vi "NotifyLvFPGACompileFinish.vi"() -> ()   [LabVIEW 2013]
uses:
  <vilib>/Utility/sysdir.llb/System Directory Type.ctl
  <vilib>/Utility/miscctls.llb/LVPointTypeDef.ctl
  <vilib>/ptbypt/NI_PtbyPt.lvlib
panel:
  out "title":string="NotifyLvFPGACompileFinish"
  in  "Prohibit time":T1
  out "smtp error msg":string
  in  "Interval_sec":i32=60
  in  "SendTo":T2
  in  "SMTP Setting":T3={"smtp server"="", "From"="", "port number"=25, "chk smtp auth"=FALSE, "userID"="", "password"="", "chk ssl"=FALSE}
  in  "Tab":enum32{"Log"}(tab)
  out "Log":string
  out "コンパイル中":bool
  out "Compile FPGA-Target":string
  out "MailBody":string
  in  "Btn SendMail":bool
  out "Compile Folder":path
  out "flag Compiling":bool
  out "監視中":bool
  out "flag Monitoring":bool
  in  "FPGA Compile path":path=path "C:/NIFPGA/compilation"
  in  "Btn Settings":bool
  in  "Btn Stop":bool
  in  "Btn Start":bool
  # "FPGAコンパイル終了時に\n指定したメールアドレスに\n結果メールを送信します。"
  # "FPGA モジュールがインストールされているPCで実行してください。"
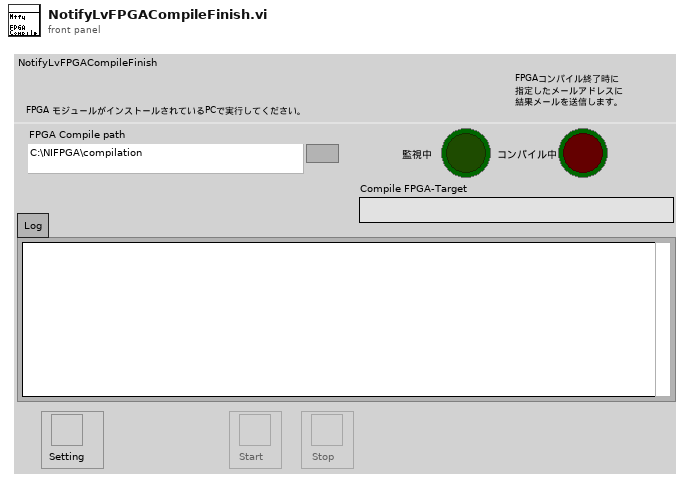
[diagram p1: front panel]
types:
  T1 = cluster{"chk enable":bool, "start hour":u8, "end hour":u8}
  T2 = cluster{"To 1":cluster{"chk":bool, "To":string}, "To 2":cluster{"chk":bool, "To":string}, "To 3":cluster{"chk":bool, "To":string}}
  T3 = cluster{"smtp server":string, "From":string, "port number":i32, "chk smtp auth":bool, "userID":string, "password":string, "chk ssl":bool}
  T4 = typedef "System Directory Type.ctl" = i32
  T5 = enum8{"Enabled", "Disabled", "Disabled and Grayed Out"}
  T6 = cluster{"SMTP Setting out":cluster{"smtp server":string, "From":string, "port number":i32, "chk smtp auth":bool, "userID":string, "password":string, "chk ssl":bool}, "SendTo out":cluster{"To 1":cluster{"chk":bool, "To":string}, "To 2":cluster{"chk":bool, "To":string}, "To 3":cluster{"chk":bool, "To":string}}, "Prohibit time out":cluster{"chk enable":bool, "start hour":u8, "end hour":u8}}
  T7 = typedef "LVPointTypeDef.ctl" = cluster{"Horizontal":i16, "Vertical":i16}
  T8 = cluster{bool, "include Ctrl key?":bool, string}[]
  T9 = cluster{"配列[0]":i16, "配列[1]":i16, "配列[2]":i16, "配列[3]":i16}
  T10 = cluster{"SMTP Setting":cluster{"smtp server":string, "From":string, "port number":i32, "chk smtp auth":bool, "userID":string, "password":string, "chk ssl":bool}, "SendTo":cluster{"To 1":cluster{"chk":bool, "To":string}, "To 2":cluster{"chk":bool, "To":string}, "To 3":cluster{"chk":bool, "To":string}}, "Prohibit time":cluster{"chk enable":bool, "start hour":u8, "end hour":u8}}
  T11 = typedef "LVRectTypeDef.ctl" = cluster{"Left":i16, "Top":i16, "Right":i16, "Bottom":i16}
  T12 = enum32{"invalid app kind", "Development System", "Run Time System", "Student Edition", "Embedded LabVIEW", "Evaluation", "Custom"}
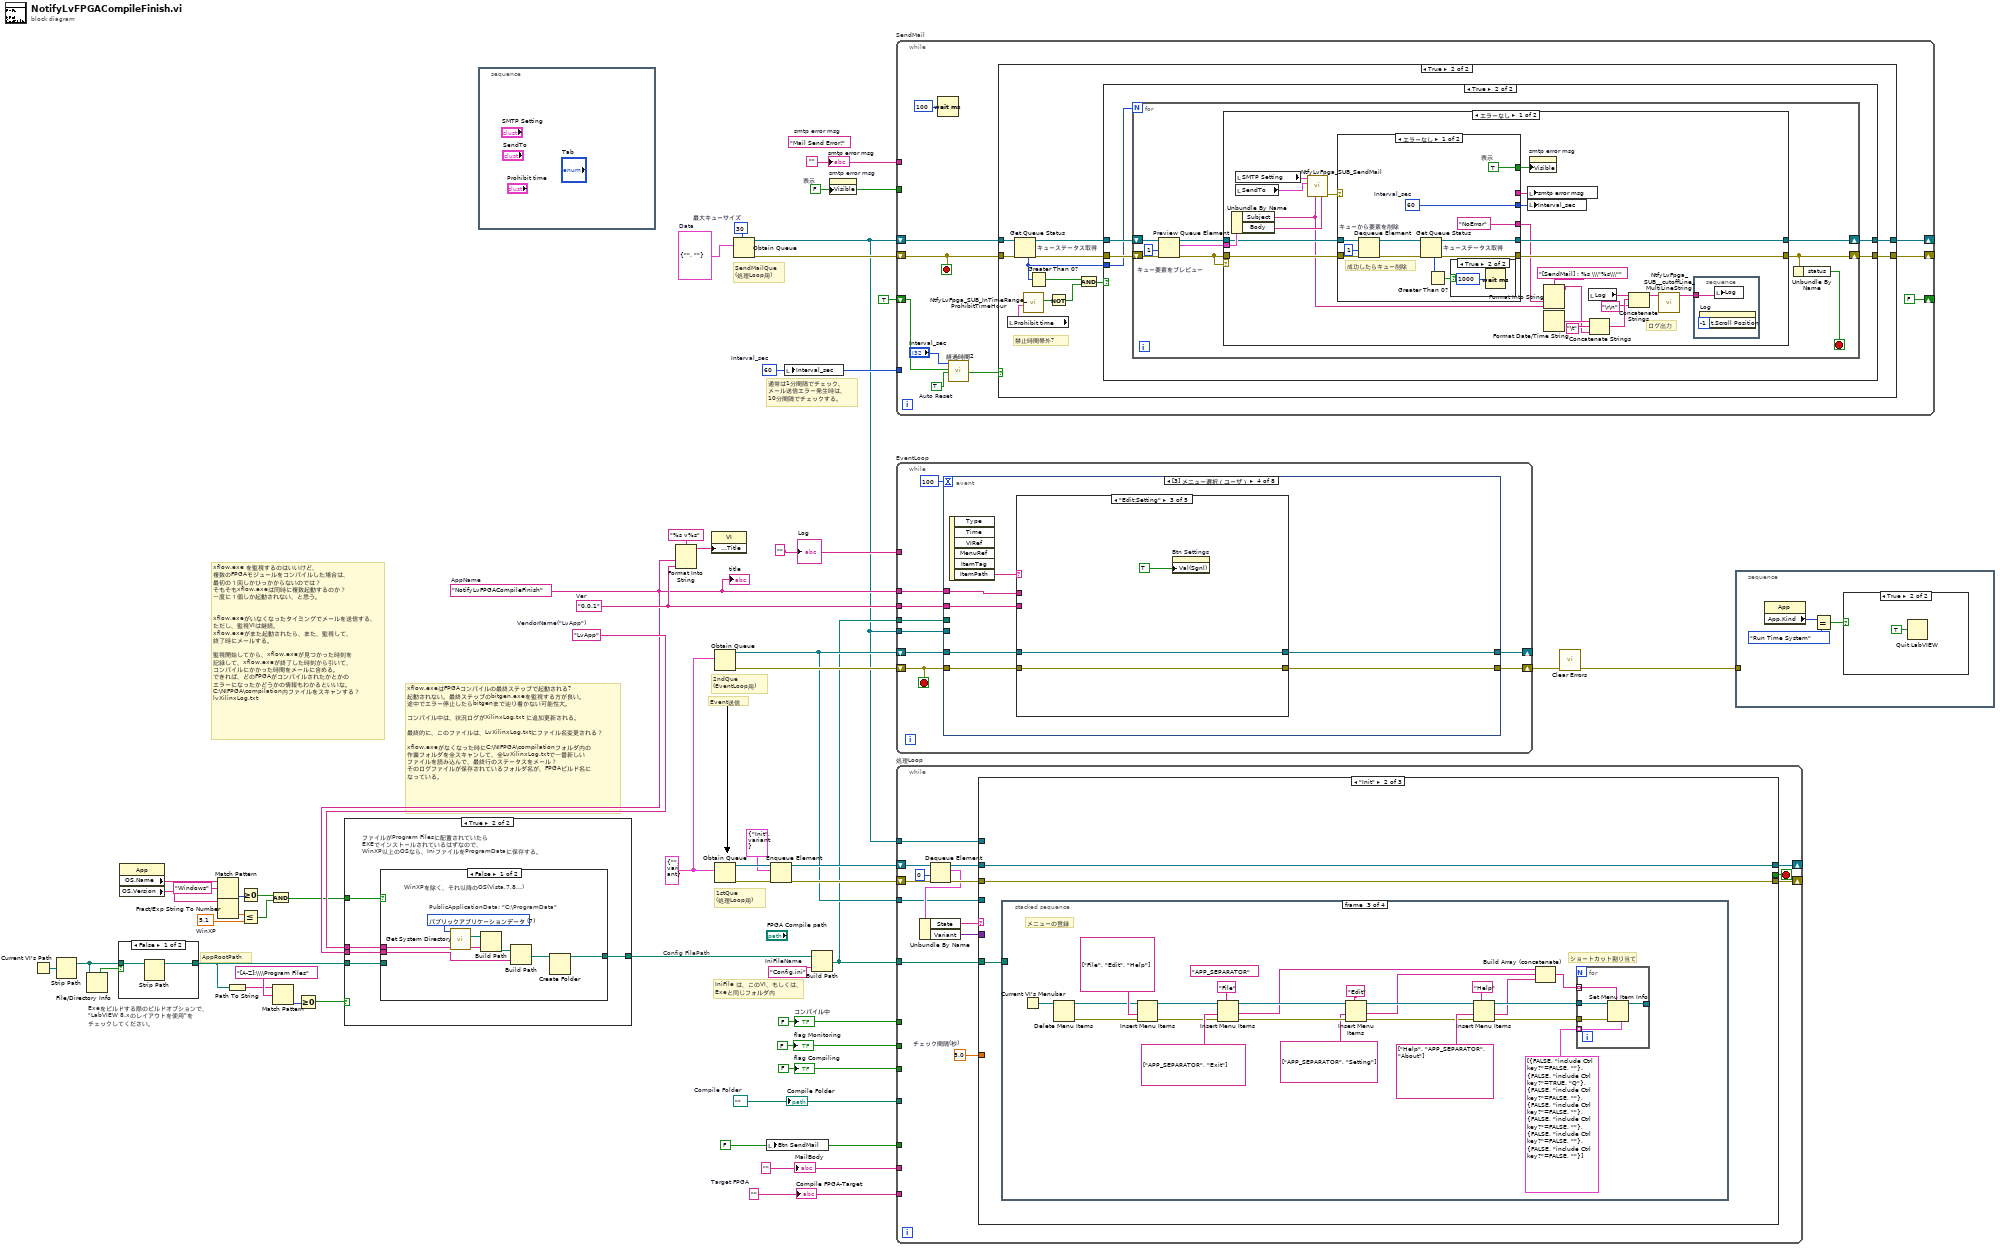
[diagram p0: block diagram]
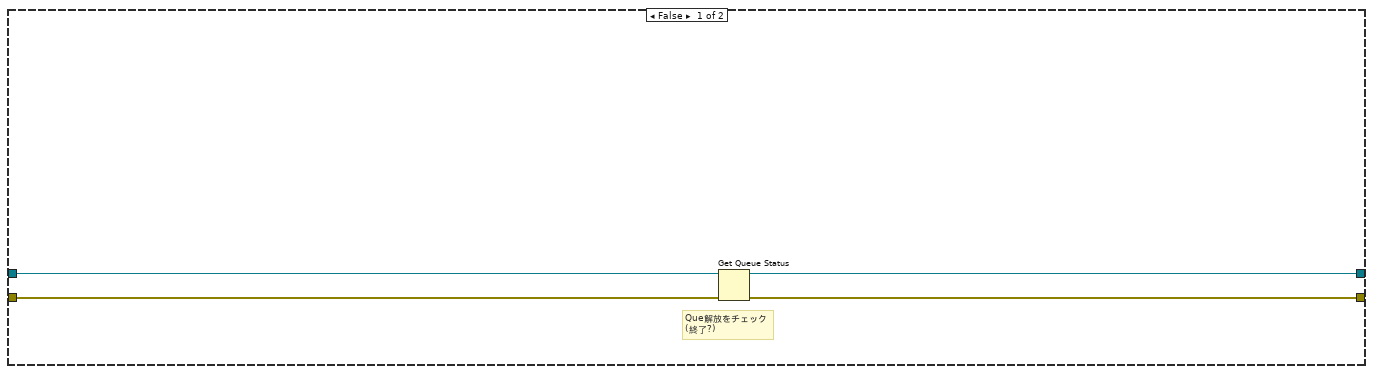
[diagram p2: hidden frame]
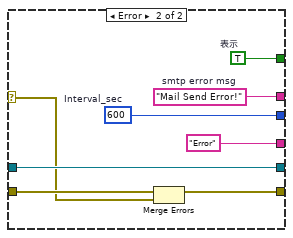
[diagram p5: hidden frame]
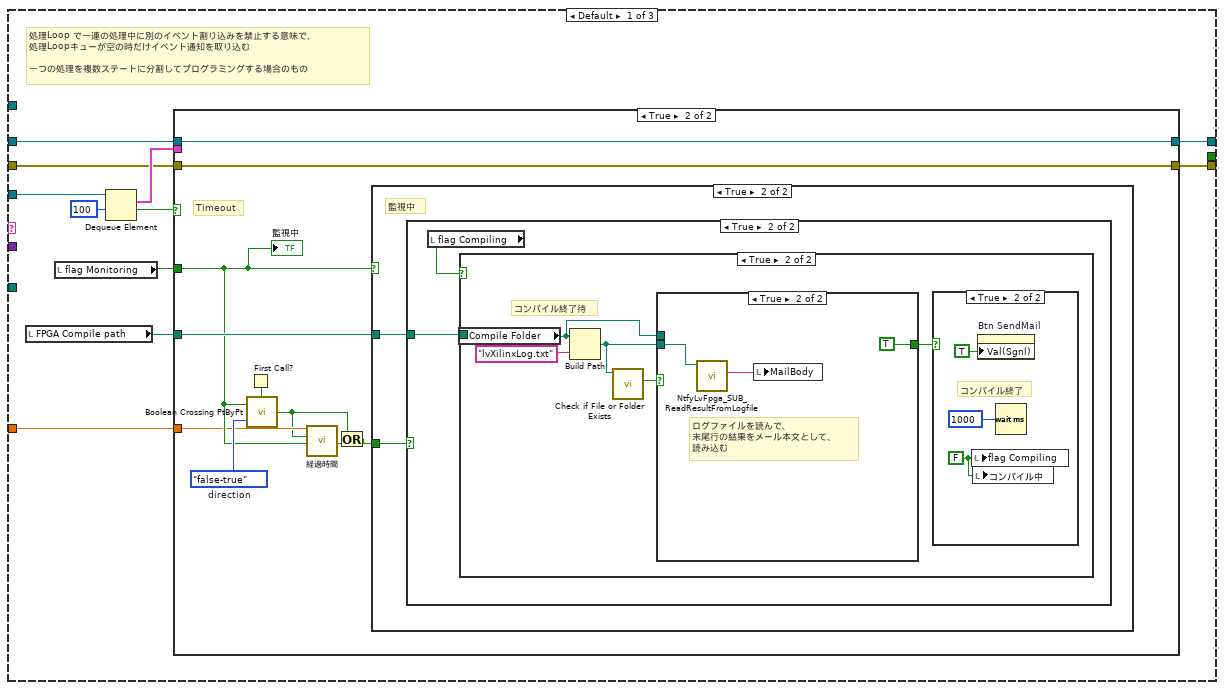
[diagram p11: hidden frame]
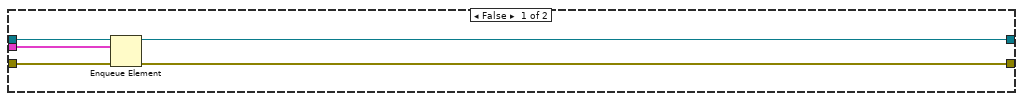
[diagram p12: hidden frame]
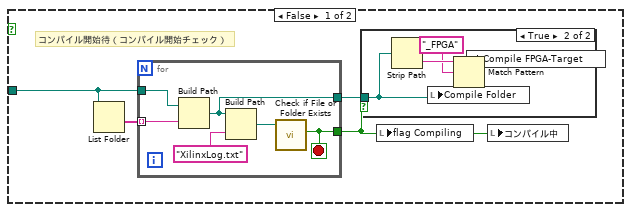
[diagram p15: hidden frame]
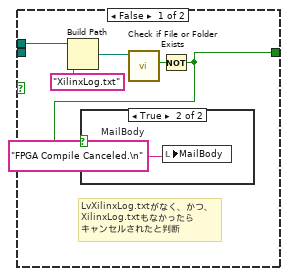
[diagram p18: hidden frame]
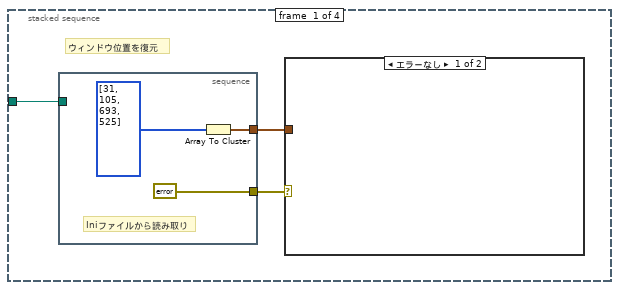
[diagram p20: hidden frame]
diagram:
  w3 = FALSE  # 表示
  w4 = ""
  (unwired) "Mail Send Error!"  # smtp error msg
  w5 = 60  # Interval_sec
  w6 = 30  # 最大キューサイズ
  w7 = cluster{"Subject":string, "Body":string} {"Subject"="", "Body"=""}  # Data
  w9 = ""
  w11 = FALSE
  w12 = ""  # Target FPGA
  w13 = ""
  w14 = FALSE
  w15 = path ""  # Compile Folder
  w16 = FALSE
  w17 = FALSE
  w28 = "LvApp"  # VendorName("LvApp")
  w33 = 5.1  # WinXP
  w38 = "Config.ini"  # IniFileName
  w41 = "0.0.1"  # Ver
  w27 = "NotifyLvFPGACompileFinish"  # AppName
  w51 = cluster{"State":string, "Variant":variant} {"State"="", "Variant"=variant}
  # "通常は1分間隔でチェック、\nメール送信エラー発生時は、\n10分間隔でチェックする。"
  # "SendMailQue\n(処理Loop用)"
  # "xflow.exeはFPGAコンパイルの最終ステップで起動される?\n起動されない。最終ステップのbitgen.exeを監視する方が良い。\n途中でエラー停止したらbitgenまで辿り着かない可能性大。\n\nコンパイル中は、状況ログがXilinxLog.txt に追加更新される。\n\n最終的に、このファイルは、LvXilinxLog.txtにファイル名変更される？\n\nxflow.exeがなくなった時にC:\\NIFPGA\\compilationフォルダ内の\n作業フォルダを全スキャンして、全LvXilinxLog.txtで一番新しい\nファイルを読み込んで、最終行のステータスをメール？\nそのログファイルが保存されているフォルダ名が、FPGAビルド名に\nなっている。"
  # "xflow.exe を監視するのはいいけど、\n複数のFPGAモジュールをコンパイルした場合は、\n最初の１回しかひっかからないのでは？\nそもそもxflow.exeは同時に複数起動するのか？\n一度に１個しか起動されない、と思う。\n\n\nxflow.exeがいなくなったタイミングでメールを送信する、\nただし、監視VIは継続。\nxflow.exeがまた起動されたら、また、監視して、\n終了時にメールする。\n\n監視開始してから、xflow.exeが見つかった時刻を\n記録して、xflow.exeが終了した時刻から引いて、\nコンパイルにかかった時間をメールに含める。\nできれば、どのFPGAがコンパイルされたかとかの\nエラーになったかどうかの情報もわかるといいな。\nC:\\NIFPGA\\compilation内ファイルをスキャンする？\nlvXilinxLog.txt"
  # "Exeをビルドする際のビルドオプションで、\n\"LabVIEW 8.xのレイアウトを使用\"を\nチェックしてください。"
  # "Config FilePath"
  # "AppRootPath"
  # "IniFile は、このVI、もしくは、\nExeと同じフォルダ内"
  # "2ndQue\n(EventLoop用)"
  # "1stQue\n(処理Loop用)"
  # "Event送信"
  n1 = Current VI's Path() -> (path=w24:path)
  n2 = Strip Path(path=w24) -> (stripped path=w25:path)  [unwired: 1 out]
  n3 = File/Directory Info(path=w25) -> (directory=w26:bool)  [unwired: 1 in, 6 out]
  n4 = case shown="FALSE" w26 {
    tunnel: w25 -> [w53 w54]
    tunnel: [w52 w54] -> w21
    frame False {
      n5 = Strip Path(path=w53) -> (stripped path=w52:path)  [unwired: 1 out]
    }
    frame True {
    }
  }
  n6 = property class="App"() -> ("OS.Name"=w37:string, "OS.Version"=w35:string)  [unwired: 2 in, 2 out]
  n7 = Match Pattern(string=w37, regular expression="Windows" ("正規表現")) -> (offset past match=w32:i32)  [unwired: 1 in, 3 out]
  n8 = Fract/Exp String To Number(string=w35) -> (number=w34:dbl)  [unwired: 3 in, 1 out]
  n9 = Path To String(path=w21) -> (string=w20:string)
  n10 = Greater Or Equal To 0?(x=w32) -> (x >= 0?=w31:bool)
  n11 = Less Or Equal?(x=w34, y=w33) -> (x <= y?=w30:bool)
  n12 = And(x=w31, y=w30) -> (x .and. y?=w23:bool)
  n13 = Match Pattern(string=w20, regular expression="[A-Z]:\\\\Program Files" ("正規表現")) -> (offset past match=w19:i32)  [unwired: 1 in, 3 out]
  n14 = Greater Or Equal To 0?(x=w19) -> (x >= 0?=w18:bool)
  n15 = case shown="TRUE" w18 {
    tunnel: w27 -> [_ w60]
    tunnel: [w55 w58] -> w29
    tunnel: w28 -> [_ w59]
    tunnel: w23 -> [_ w57]
    tunnel: w21 -> [w55 w56]
    frame False {
      # "ファイルがProgram Filesに配置されていなかったら\n開発システムでソースから実行しているか、\nExeで適当なフォルダから実行されているので、\nIniファイルは、EXE, またはTop VI と同じ場所に保存"
    }
    frame True {
      # "ファイルがProgram Filesに配置されていたら\nEXEでインストールされているはずなので、\nWinXP以上のOSなら、IniファイルをProgramDataに保存する。"
      n16 = case shown="FALSE" w57 {
        tunnel: w60 -> [w64 _]
        tunnel: w59 -> [w62 _]
        tunnel: [w61 w68] -> w58
        tunnel: w56 -> [_ w68]
        frame False {
          w67 = T4 7 items=["ユーザホーム"=0, "ユーザデスクトップ"=1, "ユーザドキュメント"=2, "ユーザアプリケーションデータ"=3, "ユーザ設定"=4, "ユーザ一時"=5, "パブリックドキュメント"=6, "パブリックアプリケーションデータ"=7, "パブリック環境設定"=8, "パブリックキャッシュ"=13, "システムコアライブラリ"=9, "システムインストールされたライブラリ"=10, "アプリケーションファイル"=11, "ブート容量ルート"=12] ("system directory type")
          # "PublicApplicationData: \"C:\\ProgramData\""
          # "WinXPを除く、それ以降のOS(Vista,7,8,..)"
          n17 = call <vilib>:"Get System Directory.vi"("system directory type"=w67) -> ("system directory"=w66:path)  [unwired: 10 in]
          n18 = Build Path(base path=w66, name or relative path=w62) -> (appended path=w65:path)
          n19 = Build Path(base path=w65, name or relative path=w64) -> (appended path=w63:path)
          n20 = Create Folder(path (use dialog)=w63) -> (created path=w61:path)  [unwired: 2 in, 2 out]
        }
        frame True {
        }
      }
    }
  }
  n21 = stacked-sequence {
    frame #0 {
    }
  }
  n22 = Format Into String(format string="%s v%s" ("形式文字列"), w27, w41) -> (resulting string=w39:string)  [unwired: 2 in, 1 out]
  n23 = property class="VI"("Front Panel.Title"=w39) -> ()  [unwired: 2 in, 2 out]
  n24 = Obtain Queue(element data type=w51) -> (queue out=w44:refnum<queue>, error out=w50:errorcluster)  [unwired: 4 in, 1 out]
  n25 = Obtain Queue(element data type=w51) -> (queue out=w49:refnum<queue>, error out=w47:errorcluster)  [unwired: 4 in, 1 out]
  n26 = Obtain Queue(max queue size (-1, unlimited)=w6, element data type=w7) -> (queue out=w1:refnum<queue>, error out=w8:errorcluster)  [unwired: 3 in, 1 out]
  n27 = local write "Btn SendMail"(w14) -> ()
  n28 = Enqueue Element(queue=w49, element=cluster{string, "バリアント":variant} {"Init", "バリアント"=variant}, error in (no error)=w47) -> (queue out=w48:refnum<queue>, error out=w46:errorcluster)  [unwired: 1 in, 1 out]
  n29 = local write "Interval_sec"(w5) -> ()
  n30 = Build Path(base path=w29, name or relative path=w38) -> (appended path=w10:path)
  n31 = property on="smtp error msg" class="Str"("Visible"=w3) -> ()  [unwired: 2 in, 2 out]
  n32 = while "SendMail" {
    shift-right: [w76] -> _
    shift-left: w1 -> [w78]
    shift-right: [w75] -> _
    shift-left: w8 -> [w77]
    tunnel: w5 -> [_]
    tunnel: w4 -> [_]
    tunnel: w3 -> [_]
    shift-right: [FALSE] -> _
    shift-left: TRUE -> [w71]
    stop <- w77 stop-if-true
    w70 = TRUE  # Auto Reset
    n33 = Wait (ms)(milliseconds to wait=u32 100) -> ()  [unwired: 1 out]
    n34 = call "経過時間2"("Time Target (s)"="Interval_sec", "Reset"=w71, "Auto Reset"=w70) -> ("Time has Elapsed"=w69:bool)  [unwired: 9 in, 7 out]
    n35 = case shown="TRUE" w69 {
      tunnel: w78 -> [w82 w94]
      tunnel: w77 -> [w81 w92]
      tunnel: [w79 w90] -> w76
      tunnel: [w80 w89] -> w75
      frame False {
        # "Que解放をチェック\n(終了?)"
        n36 = Get Queue Status(queue=w82, error in (no error)=w81) -> (queue out=w79:refnum<queue>, error out=w80:errorcluster)  [unwired: 1 in, 6 out]
      }
      frame True {
        # "禁止時間帯外?"
        n37 = local read "Prohibit time"() -> (w87:T1)
        n38 = Get Queue Status "キューステータス取得"(queue=w94, error in (no error)=w92) -> (queue out=w93:refnum<queue>, error out=w91:errorcluster, # elements in queue=w88:i32)  [unwired: 1 in, 5 out]
        n39 = call "NtfyLvFpga_SUB_InTimeRange_ProhibitTimeHour.vi"("Time Range"=w87) -> ("InRange"=w84:bool)  [unwired: 10 in]
        n40 = Greater Than 0?(x=w88) -> (x > 0?=w85:bool)
        n41 = Not(x=w84) -> (.not. x?=w83:bool)
        n42 = And(x=w85, y=w83) -> (x .and. y?=w86:bool)
        n43 = case shown="TRUE" w86 {
          tunnel: w93 -> [w96 w101]
          tunnel: w91 -> [w95 w99]
          tunnel: [w96 w100] -> w90
          tunnel: [w95 w98] -> w89
          tunnel: w88 -> [_ w97]
          frame False {
          }
          frame True {
            n44 = for {
              N: w97 -> [_]
              shift-right: [w107] -> w100
              shift-left: w101 -> [w110]
              shift-right: [w105] -> w98
              shift-left: w99 -> [w109]
              stop <- w104 stop-if-true
              n45 = Preview Queue Element "キュー要素をプレビュー"(queue=w110, timeout in ms (-1)=1, error in (no error)=w109) -> (queue out=w108:refnum<queue>, element=w103:cluster{"Subject":string, "Body":string}, error out=w106:errorcluster)  [unwired: 1 out]
              n46 = case shown="エラーなし" w106 {
                tunnel: w108 -> [w127 w158]
                tunnel: [w125 w158] -> w107
                tunnel: w106 -> [w126 w157]
                tunnel: [w124 w157] -> w105
                tunnel: w103 -> [w129 _]
                frame No Error {
                  # "ログ出力"
                  n47 = Unbundle By Name(w129) -> ("Subject"=w114:string, "Body"=w128:string)
                  n48 = local read "SMTP Setting"() -> (w132:T3)
                  n49 = local read "SendTo"() -> (w133:T2)
                  n50 = call "NtfyLvFpga_SUB_SendMail.vi"("Body"=w128, "Subject"=w114, "SendTo"=w133, "SMTP Setting"=w132) -> ("error out"=w131:errorcluster)  [unwired: 7 in]
                  n51 = case shown="エラーなし" w131 {
                    selector: w131 -> [_ w152]
                    tunnel: [w147 w156] -> w130
                    tunnel: w127 -> [w146 w155]
                    tunnel: w126 -> [w145 w154]
                    tunnel: [w139 w155] -> w125
                    tunnel: [w138 w153] -> w124
                    tunnel: [_ w151] -> w123
                    tunnel: [w143 w150] -> w122
                    tunnel: ["NoError" "Error"] -> w113
                    frame No Error {
                      w143 = TRUE  # 表示
                      w147 = 60  # Interval_sec
                      # "成功したらキュー削除"
                      n52 = Dequeue Element "キューから要素を削除"(queue=w146, timeout in ms (-1)=1, error in (no error)=w145) -> (queue out=w141:refnum<queue>, error out=w140:errorcluster)  [unwired: 2 out]
                      n53 = Get Queue Status "キューステータス取得"(queue=w141, error in (no error)=w140) -> (queue out=w139:refnum<queue>, error out=w138:errorcluster, # elements in queue=w137:i32)  [unwired: 1 in, 5 out]
                      n54 = Greater Than 0?(x=w137) -> (x > 0?=w136:bool)
                      n55 = case shown="TRUE" w136 {
                        frame False {
                        }
                        frame True {
                          n56 = Wait (ms)(milliseconds to wait=u32 1000) -> ()  [unwired: 1 out]
                        }
                      }
                    }
                    frame Error {
                      w150 = TRUE  # 表示
                      w151 = "Mail Send Error!"  # smtp error msg
                      w156 = 600  # Interval_sec
                      n57 = Merge Errors(w154, w152) -> (w153:errorcluster)
                    }
                  }
                  n58 = local write "smtp error msg"(w123) -> ()
                  n59 = local write "Interval_sec"(w130) -> ()
                  n60 = property on="smtp error msg" class="Str"("Visible"=w122) -> ()  [unwired: 2 in, 2 out]
                  n61 = Format Into String(format string="[SendMail] : %s \\\"%s\\\"", w113, w114) -> (resulting string=w111:string)  [unwired: 2 in, 1 out]
                  n62 = Format Date/Time String() -> (date/time string=w116:string)  [unwired: 3 in]
                  n63 = local read "Log"() -> (w120:string)
                  n64 = Concatenate Strings(w116, "\t", w111) -> (w121:string)
                  n65 = Concatenate Strings(w120, w121, "\r\n") -> (w119:string)
                  n66 = call "NtfyLvFpga_SUB__cutoffLine_MultiLineString.vi"("String"=w119) -> ("String out"=w118:string)  [unwired: 10 in]
                  n67 = stacked-sequence {
                    tunnel: w118 -> [w134]
                    frame #0 {
                      n68 = property on="Log" class="Str"("Text.Scroll Position"=-1) -> ()  [unwired: 2 in, 2 out]
                      n69 = local write "Log"(w134) -> ()
                    }
                  }
                }
                frame Error {
                }
              }
              n70 = Unbundle By Name(w105) -> ("status"=w104:bool)
            }
          }
        }
      }
    }
  }
  n71 = while "EventLoop" {
    shift-right: [w165] -> _
    shift-left: w44 -> [w166]
    shift-right: [w164] -> w43
    shift-left: w50 -> [w163]
    tunnel: w27 -> [w162]
    tunnel: w41 -> [w161]
    tunnel: w10 -> [w160]
    tunnel: w9 -> [_]
    tunnel: w1 -> [w159]
    stop <- w163 stop-if-true
    n72 = event shown="[3] メニュー選択（ユーザ）" {
      selector: _ -> [_ _ _ _ _ _ _ _]
      dyn-events: _ -> [_ _ _ _ _ _ _ _]
      timeout: 100 -> [_ _ _ _ _ _ _ _]
      tunnel: w166 -> [w171 w177 w183 w191 w217 w225 w245 w267]
      tunnel: [w168 w176 w182 w190 w217 w225 w245 w267] -> w165
      tunnel: w163 -> [w170 w175 w181 w189 w216 w224 w244 w266]
      tunnel: [w169 w174 w180 w188 w216 w224 w244 w266] -> w164
      tunnel: w162 -> [_ _ _ w186 _ _ _ _]
      tunnel: w161 -> [_ _ _ w185 _ _ _ _]
      tunnel: w160 -> [_ _ _ _ _ _ _ w262]
      tunnel: w159 -> [_ _ _ _ _ w218 w231 _]
      event Timeout {
        # "EventLoopの終了用"
        # "Que解放をチェック\n(終了?)"
        n73 = event-data() -> ()  [unwired: 1 in, 2 out]
        n74 = Get Queue Status(queue=w171, error in (no error)=w170) -> (queue out=w168:refnum<queue>, error out=w169:errorcluster)  [unwired: 1 in, 6 out]
      }
      event Application Instance Close? {
        n75 = event-data() -> ()  [unwired: 1 in, 4 out]
        n76 = Enqueue Element(queue=w177, element=cluster{string, "バリアント":variant} {"Final", "バリアント"=variant}, error in (no error)=w175) -> (queue out=w176:refnum<queue>, error out=w174:errorcluster)  [unwired: 1 in, 1 out]
        n77 = event-data("SilentShutdown"=TRUE, "Discard?"=FALSE ("破棄?")) -> ()  [unwired: 1 in, 1 out]
      }
      event Panel Close? {
        n78 = event-data() -> ()  [unwired: 1 in, 3 out]
        n79 = Enqueue Element(queue=w183, element=cluster{string, "バリアント":variant} {"Final", "バリアント"=variant}, error in (no error)=w181) -> (queue out=w182:refnum<queue>, error out=w180:errorcluster)  [unwired: 1 in, 1 out]
        n80 = event-data("Discard?"=TRUE) -> ()  [unwired: 1 in, 1 out]
      }
      event Menu Selection (User) {
        n81 = event-data() -> ("ItemPath"=w187:string)  [unwired: 1 in, 5 out]
        n82 = case shown="\"Edit:Setting\"" w187 {
          tunnel: w191 -> [w193 w198 w201 w207 w209]
          tunnel: [w193 w197 w201 w207 w209] -> w190
          tunnel: w189 -> [w192 w196 w200 w206 w208]
          tunnel: [w192 w195 w200 w206 w208] -> w188
          tunnel: w186 -> [_ _ _ w205 _]
          tunnel: w185 -> [_ _ _ w204 _]
          frame Default {
          }
          frame "File:Exit" {
            n83 = Enqueue Element(queue=w198, element=cluster{string, "バリアント":variant} {"Final", "バリアント"=variant}, error in (no error)=w196) -> (queue out=w197:refnum<queue>, error out=w195:errorcluster)  [unwired: 1 in, 1 out]
          }
          frame "Edit:Setting" {
            n84 = property on="Btn Settings" class="Bool （指定）"("Val(Sgnl)"=TRUE) -> ()  [unwired: 2 in, 2 out]
          }
          frame "Help:About" {
            n85 = Format Into String(format string="%s\n\nVersion : %s" ("メッセージ"), w205, w204) -> (resulting string=w202:string)  [unwired: 2 in, 1 out]
            n86 = One Button Dialog(message=w202) -> ()  [unwired: 1 in, 1 out]
          }
          frame "Help:Help" {
          }
        }
      }
      event "Btn Start": Value Change {
        w212 = FALSE ("flag Compiling")
        n87 = event-data() -> ()  [unwired: 1 in, 5 out]
        n88 = local write "Compile FPGA-Target"("") -> ()
        n89 = local write "Compile Folder"(path "") -> ()
        n90 = local write "flag Monitoring"(TRUE) -> ()
        n91 = local write "flag Compiling"(w212) -> ()
        n92 = local write "コンパイル中"(w212) -> ()
        n93 = property on="Btn Stop" class="Bool"("DisabledEnum"=T5."Enabled") -> ()  [unwired: 2 in, 2 out]
        n94 = property on="Btn Start" class="Bool"("DisabledEnum"=T5."Disabled and Grayed Out") -> ()  [unwired: 2 in, 2 out]
      }
      event "Btn Stop": Value Change {
        w221 = FALSE ("flag Compiling")
        # "たまったメール送信\nデータをすべて削除"
        n95 = event-data() -> ()  [unwired: 1 in, 5 out]
        n96 = Flush Queue(queue=w218) -> ()  [unwired: 1 in, 3 out]
        n97 = local write "Compile Folder"(path "") -> ()
        n98 = local write "flag Monitoring"(FALSE) -> ()
        n99 = local write "コンパイル中"(w221) -> ()
        n100 = local write "flag Compiling"(w221) -> ()
        n101 = property on="Btn Stop" class="Bool"("DisabledEnum"=T5."Disabled and Grayed Out") -> ()  [unwired: 2 in, 2 out]
        n102 = property on="Btn Start" class="Bool"("DisabledEnum"=T5."Enabled") -> ()  [unwired: 2 in, 2 out]
      }
      event "Btn SendMail": Value Change {
        # "メールデータをキュー送信"
        # "ログ出力"
        # "GetHostname"
        n103 = event-data() -> ()  [unwired: 1 in, 5 out]
        n104 = String To IP() -> (0:w241:u32)  [unwired: 1 in]
        n105 = local read "Compile FPGA-Target"() -> (w232:string)
        n106 = IP To String(2:w241) -> (0:w234:string)  [unwired: 1 in]
        n107 = local write "Btn SendMail"(FALSE) -> ()
        n108 = Match Pattern(string=w234, regular expression="\\.") -> (before substring=w233:string)  [unwired: 1 in, 3 out]
        n109 = local read "MailBody"() -> (w229:string)
        n110 = Format Into String(format string="[FPGA Compile Finish]  %s on %s", w232, w233) -> (resulting string=w230:string)  [unwired: 2 in, 1 out]
        n111 = Bundle(w230, "MailBody"=w229) -> (w228:cluster{string, "MailBody":string})  [unwired: 1 in]
        n112 = Enqueue Element(queue=w231, element=w228, timeout in ms (-1)=1) -> (error out=w226:errorcluster)  [unwired: 1 in, 2 out]
        n113 = stacked-sequence {
          tunnel: [w252] -> w237
          tunnel: w233 -> [w248]
          tunnel: w232 -> [w247]
          tunnel: w226 -> [_]
          frame #0 {
            n114 = Format Into String(format string="%s on %s", w247, w248) -> (resulting string=w246:string)  [unwired: 2 in, 1 out]
            n115 = Format Date/Time String() -> (date/time string=w254:string)  [unwired: 3 in]
            n116 = Concatenate Strings("[FPGA Compile Finish] : ", w246) -> (w250:string)
            n117 = Concatenate Strings(w254, "\t", w250) -> (w252:string)
          }
        }
        n118 = local read "Log"() -> (w240:string)
        n119 = Concatenate Strings(w240, w237, "\r\n") -> (w239:string)
        n120 = call "NtfyLvFpga_SUB__cutoffLine_MultiLineString.vi"("String"=w239) -> ("String out"=w238:string)  [unwired: 10 in]
        n121 = stacked-sequence {
          tunnel: w238 -> [w255]
          frame #0 {
            n122 = property on="Log" class="Str"("Text.Scroll Position"=-1) -> ()  [unwired: 2 in, 2 out]
            n123 = local write "Log"(w255) -> ()
          }
        }
      }
      event "Btn Settings": Value Change {
        n124 = event-data() -> ()  [unwired: 1 in, 1 out]
        n125 = local read "SMTP Setting"() -> (w261:T3)
        n126 = local read "Prohibit time"() -> (w258:T1)
        n127 = local read "SendTo"() -> (w260:T2)
        n128 = local write "Btn Settings"(FALSE) -> ()
        n129 = call "NtfyLvFpga_SUB_SettingPanel.vi"("Prohibit time"=w258, "SendTo"=w260, "SMTP Setting"=w261) -> ("Prohibit time out"=w259:T1, "OK?"=w265:bool, "SendTo out"=w264:T2, "SMTP Setting out"=w263:T3)  [unwired: 5 in]
        n130 = case shown="TRUE" w265 {
          tunnel: w264 -> [_ w271]
          tunnel: w263 -> [_ w272]
          tunnel: w262 -> [_ w273]
          tunnel: w261 -> [_ w278]
          tunnel: w260 -> [_ w277]
          tunnel: w259 -> [_ w268]
          tunnel: w258 -> [_ w270]
          frame False {
          }
          frame True {
            # "OK"
            n131 = Not Equal?(x=w272, y=w278) -> (x != y?=w276:bool)
            n132 = Not Equal?(x=w271, y=w277) -> (x != y?=w275:bool)
            n133 = local write "SMTP Setting"(w272) -> ()
            n134 = local write "SendTo"(w271) -> ()
            n135 = local write "Prohibit time"(w268) -> ()
            n136 = Not Equal?(x=w268, y=w270) -> (x != y?=w269:bool)
            n137 = Compound Arithmetic op=OR(w276, w275, w269) -> (w274:bool)
            n138 = case shown="TRUE" w274 {
              tunnel: w273 -> [_ w285]
              tunnel: w272 -> [_ w288]
              tunnel: w271 -> [_ w287]
              tunnel: w268 -> [_ w279]
              frame False {
              }
              frame True {
                w286 = TRUE  # Write(T)
                # "Update IniFile"
                n139 = Bundle("SMTP Setting out"=w288, "SendTo out"=w287, "Prohibit time out"=w279) -> (w284:T6)  [unwired: 1 in]
                n140 = call "NtfyLvFpga_SUB_ValidationSmtpConfig.vi"("Config"=w284) -> ("Valid?"=w283:bool)  [unwired: 10 in]
                n141 = call "NtfyLvFpga_SUB_ReadWriteConfigIni.vi"("Read/Write(T)"=w286, "Config"=w284, "ConfigIni filepath"=w285) -> ()  [unwired: 7 in, 2 out]
                n142 = Select(t=T5."Enabled", s=w283, f=T5."Disabled and Grayed Out") -> (s? t:f=w282:T5)
                n143 = property on="Btn Start" class="Bool"("DisabledEnum"=w282) -> ()  [unwired: 2 in, 2 out]
              }
            }
          }
        }
      }
    }
  }
  n144 = while "処理Loop" {
    shift-right: [w298] -> _
    shift-left: w48 -> [w303]
    shift-right: [w297] -> _
    shift-left: w46 -> [w300]
    tunnel: w44 -> [w293]
    tunnel: w10 -> [w291]
    tunnel: w17 -> [_]
    tunnel: w16 -> [_]
    tunnel: w15 -> [_]
    tunnel: w14 -> [_]
    tunnel: w13 -> [_]
    tunnel: w12 -> [_]
    tunnel: w11 -> [_]
    tunnel: w1 -> [w289]
    stop <- w292 stop-if-true
    w290 = 5.0  # チェック間隔(秒)
    n145 = Dequeue Element(queue=w303, timeout in ms (-1)=0 ("タイムアウト（ms）（-1）"), error in (no error)=w300) -> (queue out=w302:refnum<queue>, element=w296:cluster{"State":string, "Variant":variant}, error out=w299:errorcluster)  [unwired: 1 out]
    n146 = Unbundle By Name(w296) -> ("State"=w295:string, "Variant"=w294:variant)
    n147 = case shown="\"Init\"" w295 {
      tunnel: w302 -> [w311 w367 w437]
      tunnel: w293 -> [w314 _ w435]
      tunnel: w299 -> [w309 w366 w434]
      tunnel: [w310 w367 refnum<queue> refnum ("queue out")] -> w298
      tunnel: [w308 w366 w433] -> w297
      tunnel: w294 -> [_ _ _]
      tunnel: [_ _ TRUE] -> w292
      tunnel: w291 -> [_ w365 w432]
      tunnel: w290 -> [w304 _ _]
      tunnel: w289 -> [_ _ w431]
      frame Default {
        # "処理Loop で一連の処理中に別のイベント割り込みを禁止する意味で、\n処理Loopキューが空の時だけイベント通知を取り込む\n\n一つの処理を複数ステートに分割してプログラミングする場合のもの"
        n148 = local read "FPGA Compile path"() -> (w305:path)
        n149 = local read "flag Monitoring"() -> (w306:bool)
        n150 = Dequeue Element(queue=w314, timeout in ms (-1)=100 ("タイムアウト（ms）（-1）")) -> (element=w312:cluster{"State":string, "Variant":variant}, timed out?=w307:bool)  [unwired: 1 in, 2 out]
        n151 = case shown="TRUE" w307 {
          tunnel: w312 -> [w319 _]
          tunnel: w311 -> [w318 w329]
          tunnel: [w317 w329] -> w310
          tunnel: w309 -> [w316 w328]
          tunnel: [w315 w328] -> w308
          tunnel: w306 -> [_ w325]
          tunnel: w305 -> [_ w327]
          tunnel: w304 -> [_ w323]
          frame False {
            n152 = Enqueue Element(queue=w318, element=w319, error in (no error)=w316) -> (queue out=w317:refnum<queue>, error out=w315:errorcluster)  [unwired: 1 in, 1 out]
          }
          frame True {
            w326 = enum16{"either", "false-true", "true-false"}."false-true"  # direction
            # "Timeout"
            n153 = First Call?() -> (First Call?: T/F=w324:bool)
            n154 = call <vilib>:"Boolean Crossing PtByPt.vi"("initialize"=w324, "direction"=w326, "input"=w325) -> ("crossing"=w321:bool)
            n155 = call "経過時間"("Time Target (s)"=w323, "Reset"=w321, "Auto Reset"=w325) -> ("Time has Elapsed"=w322:bool)  [unwired: 9 in, 7 out]
            n156 = Or(x=w321, y=w322) -> (x .or. y?=w320:bool)
            n157 = case shown="TRUE" w325 {
              tunnel: w327 -> [_ w330]
              tunnel: w320 -> [_ w331]
              frame False {
                # "idle 中"
              }
              frame True {
                # "監視中"
                n158 = case shown="TRUE" w331 {
                  tunnel: w330 -> [_ w333]
                  frame False {
                  }
                  frame True {
                    n159 = local read "flag Compiling"() -> (w332:bool)
                    n160 = case shown="TRUE" w332 {
                      tunnel: w333 -> [w336 _]
                      frame False {
                        # "コンパイル開始待（コンパイル開始チェック）"
                        n161 = List Folder(path=w336) -> (folder names=w337:string[])  [unwired: 3 in, 3 out]
                        n162 = for {
                          tunnel: w337 -> [w346] mode=indexing
                          tunnel: w336 -> [w347]
                          tunnel: [w343] -> w334
                          tunnel: [w342] -> w335
                          stop <- w343 stop-if-true
                          n163 = Build Path(base path=w347, name or relative path=w346) -> (appended path=w342:path)
                          n164 = Build Path(base path=w342, name or relative path="XilinxLog.txt") -> (appended path=w344:path)
                          n165 = call <vilib>:"Check if File or Folder Exists.vi"("path"=w344) -> ("file or folder exists?"=w343:bool)  [unwired: 8 in, 2 out]
                        }
                        n166 = case shown="TRUE" w334 {
                          tunnel: w335 -> [_ w339]
                          frame False {
                          }
                          frame True {
                            n167 = Strip Path(path=w339) -> (name=w341:string)  [unwired: 1 out]
                            n168 = local write "Compile Folder"(w339) -> ()
                            n169 = Match Pattern(string=w341, regular expression="_FPGA") -> (before substring=w338:string)  [unwired: 1 in, 3 out]
                            n170 = local write "Compile FPGA-Target"(w338) -> ()
                          }
                        }
                        n171 = local write "flag Compiling"(w334) -> ()
                        n172 = local write "コンパイル中"(w334) -> ()
                      }
                      frame True {
                        # "コンパイル終了待"
                        n173 = local read "Compile Folder"() -> (w348:path)
                        n174 = Build Path(base path=w348, name or relative path="lvXilinxLog.txt") -> (appended path=w350:path)
                        n175 = call <vilib>:"Check if File or Folder Exists.vi"("path"=w350) -> ("file or folder exists?"=w351:bool)  [unwired: 8 in, 2 out]
                        n176 = case shown="TRUE" w351 {
                          tunnel: [w356 TRUE] -> w349
                          tunnel: w350 -> [_ w363]
                          tunnel: w348 -> [w360 _]
                          frame False {
                            # "LvXilinxLog.txtがなく、かつ、\nXilinxLog.txtもなかったら\nキャンセルされたと判断"
                            n177 = Build Path(base path=w360, name or relative path="XilinxLog.txt") -> (appended path=w358:path)
                            n178 = call <vilib>:"Check if File or Folder Exists.vi"("path"=w358) -> ("file or folder exists?"=w357:bool)  [unwired: 8 in, 2 out]
                            n179 = Not(x=w357) -> (.not. x?=w356:bool)
                            n180 = case shown="TRUE" w356 {
                              frame False {
                              }
                              frame True {
                                w361 = "FPGA Compile Canceled.\n"  # MailBody
                                n181 = local write "MailBody"(w361) -> ()
                              }
                            }
                          }
                          frame True {
                            # "ログファイルを読んで、\n末尾行の結果をメール本文として、\n読み込む"
                            n182 = call "NtfyLvFpga_SUB_ReadResultFromLogfile.vi"("filepath"=w363) -> ("UTF8 TEXT"=w362:string)  [unwired: 9 in, 1 out]
                            n183 = local write "MailBody"(w362) -> ()
                          }
                        }
                        n184 = case shown="TRUE" w349 {
                          frame False {
                          }
                          frame True {
                            w353 = FALSE
                            # "コンパイル終了"
                            n185 = local write "flag Compiling"(w353) -> ()
                            n186 = local write "コンパイル中"(w353) -> ()
                            n187 = property on="Btn SendMail" class="Bool （指定）"("Val(Sgnl)"=TRUE) -> ()  [unwired: 2 in, 2 out]
                            n188 = Wait (ms)(milliseconds to wait=u32 1000) -> ()  [unwired: 1 out]
                          }
                        }
                      }
                    }
                  }
                }
              }
            }
            "監視中" <- w325
          }
        }
      }
      frame "Init" {
        n189 = stacked-sequence {
          tunnel: w365 -> [w368 _ _ w422]
          frame #0 {
            # "ウィンドウ位置を復元"
            n190 = stacked-sequence {
              tunnel: [w371] -> w370
              tunnel: [errorcluster {"status"=FALSE, "code"=0, "source"=""} ("error in (no error)")] -> w369
              tunnel: w368 -> [_]
              frame #0 {
                # "Iniファイルから読み取り"
                n191 = Array To Cluster(array=i16[] [31, 105, 693, 525] ("配列")) -> (cluster=w371:T9)
              }
            }
            n192 = case shown="エラーなし" w369 {
              tunnel: w370 -> [_ _]
              frame No Error {
              }
              frame Error {
              }
            }
          }
          frame #1 {
            # "パネルの位置を原点に戻す"
            n193 = property class="VI"() -> (reference out=w377:refnum<vi>, error out=w380:errorcluster, "Panel"=w374:refnum<vi>)  [unwired: 2 in]
            n194 = property on="プロパティノード" class="パネル"(reference=w374, error in=w380) -> (reference out=w376:refnum<vi>, "Panes[]"=w375:refnum<vi>[])  [unwired: 1 out]
            n195 = for {
              tunnel: w375 -> [w385] mode=indexing
              tunnel: [w382] -> w378
              # "基点(0, 0)"
              n196 = property on="プロパティノード" class="ペーン"(reference=w385, "Origin"=T7 {"Horizontal"=0, "Vertical"=0} ("原点")) -> (reference out=w384:refnum<vi>, error out=w383:errorcluster)  [unwired: 1 in]
              n197 = Close Reference(reference=w384, error in (no error)=w383) -> (error out=w382:errorcluster)
            }
            n198 = Close Reference(reference=w376, error in (no error)=w378) -> (error out=w379:errorcluster)
            n199 = Close Reference(reference=w377, error in (no error)=w379) -> ()  [unwired: 1 out]
          }
          frame #2 {
            (unwired) "APP_SEPARATOR"
            # "ショートカット割り当て"
            # "メニューの登録"
            n200 = Current VI's Menubar() -> (w400:refnum<k9>)
            n201 = Delete Menu Items(9:w400) -> (0:w402:errorcluster, 3:w401:refnum<k9>)  [unwired: 3 in]
            n202 = Insert Menu Items(6:w402, 7:string[] ["File", "Edit", "Help"] ("item tags"), 9:w401) -> (0:w406:errorcluster, 3:w405:refnum<k9>)  [unwired: 3 in, 1 out]
            n203 = Insert Menu Items(5:"File" ("menu tag"), 6:w406, 7:string[] ["APP_SEPARATOR", "Exit"] ("item tags"), 9:w405) -> (0:w390:errorcluster, 1:w395:string[], 3:w408:refnum<k9>)  [unwired: 2 in]
            n204 = Insert Menu Items(5:"Edit" ("menu tag"), 6:w390, 7:string[] ["APP_SEPARATOR", "Setting"] ("item tags"), 9:w408) -> (0:w389:errorcluster, 1:w388:string[], 3:w391:refnum<k9>)  [unwired: 2 in]
            n205 = Insert Menu Items(5:"Help" ("menu tag"), 6:w389, 7:string[] ["Help", "APP_SEPARATOR", "About"] ("item tags"), 9:w391) -> (0:w396:errorcluster, 1:w394:string[], 3:w397:refnum<k9>)  [unwired: 2 in]
            n206 = Build Array (concatenate)(w395, w388, w394) -> (w392:string[])
            n207 = for {
              tunnel: w397 -> [w413]
              tunnel: w396 -> [w412]
              tunnel: [w411] -> _
              tunnel: T8 [{FALSE, "include Ctrl key?"=FALSE, ""}, {FALSE, "include Ctrl key?"=TRUE, "Q"}, {FALSE, "include Ctrl key?"=FALSE, ""}, {FALSE, "include Ctrl key?"=FALSE, ""}, {FALSE, "include Ctrl key?"=FALSE, ""}, {FALSE, "include Ctrl key?"=FALSE, ""}, {FALSE, "include Ctrl key?"=FALSE, ""}] -> [w410] mode=indexing
              tunnel: w392 -> [w409] mode=indexing
              n208 = Set Menu Item Info(4:w410, 7:w409, 8:w412, 11:w413) -> (3:w411:refnum<k9>)  [unwired: 3 in, 1 out]
            }
          }
          frame #3 {
            w423 = FALSE  # Read(F)
            # "パネル制御器の初期化"
            n209 = call "NtfyLvFpga_SUB_ReadWriteConfigIni.vi"("Read/Write(T)"=w423, "ConfigIni filepath"=w422) -> ("error out"=w421:errorcluster, "Config out"=w420:T10)  [unwired: 8 in]
            n210 = case shown="エラーなし" w421 {
              tunnel: w420 -> [w429 _]
              tunnel: [w425 _] -> w416
              frame No Error {
                n211 = Unbundle By Name(w429) -> ("SMTP Setting"=w428:T3, "SendTo"=w427:T2, "Prohibit time"=w424:T1)
                n212 = local write "SMTP Setting"(w428) -> ()
                n213 = local write "SendTo"(w427) -> ()
                n214 = Bundle("SMTP Setting"=w428, "SendTo"=w427, "Prohibit time"=w424) -> (w426:T10)  [unwired: 1 in]
                n215 = call "NtfyLvFpga_SUB_ValidationSmtpConfig.vi"("Config"=w426) -> ("Valid?"=w425:bool)  [unwired: 10 in]
                n216 = local write "Prohibit time"(w424) -> ()
              }
              frame Error {
                n217 = One Button Dialog(message="Settingボタンを押して、\nメール送信設定を\nしてください。") -> ()  [unwired: 1 in, 1 out]
              }
            }
            n218 = Select(t=T5."Enabled", s=w416, f=T5."Disabled and Grayed Out") -> (s? t:f=w415:T5)
            n219 = property on="Btn Stop" class="Bool"("DisabledEnum"=T5."Disabled and Grayed Out") -> ()  [unwired: 2 in, 2 out]
            n220 = property on="Btn Start" class="Bool"("DisabledEnum"=w415) -> ()  [unwired: 2 in, 2 out]
            n221 = property on="Btn Settings" class="Bool （指定）"("DisabledEnum"=T5."Enabled") -> ()  [unwired: 2 in, 2 out]
          }
        }
      }
      frame "Final" {
        n222 = stacked-sequence {
          tunnel: w432 -> [w440 _]
          frame #0 {
            n223 = property class="VI"() -> ("Front Panel.PanelBounds"=w439:T11)  [unwired: 2 in, 2 out]
            n224 = stacked-sequence {
              tunnel: w440 -> [_]
              tunnel: w439 -> [w441]
              frame #0 {
                # "現在のWindow位置を\nIniファイルに保存"
                n225 = Cluster To Array(cluster=w441) -> ()  [unwired: 1 out]
              }
            }
          }
          frame #1 {
            w442 = FALSE
            n226 = local write "監視中"(w442) -> ()
            n227 = local write "コンパイル中"(w442) -> ()
          }
        }
        n228 = Release Queue(queue=w431) -> ()  [unwired: 2 in, 3 out]
        n229 = Release Queue(queue=w437, error in (no error)=w434) -> (error out=w433:errorcluster)  [unwired: 1 in, 2 out]
        n230 = Release Queue(queue=w435) -> ()  [unwired: 2 in, 3 out]
      }
    }
  }
  n231 = call <vilib>:"Clear Errors.vi"("error in (no error)"=w43) -> ("error out"=w42:errorcluster)  [unwired: 6 in]
  n232 = stacked-sequence {
    tunnel: w42 -> [_]
    frame #0 {
      n233 = property class="App"() -> ("App.Kind"=w445:T12)  [unwired: 2 in, 2 out]
      n234 = Equal?(x=w445, y=T12."Run Time System" ("アプリケーション:種類")) -> (x = y?=w443:bool)
      n235 = case shown="TRUE" w443 {
        frame False {
        }
        frame True {
          n236 = Quit LabVIEW(quit? (T)=TRUE ("終了?（T）")) -> ()
        }
      }
    }
  }
  "title" <- w27
  "flag Monitoring" <- w17
  "flag Compiling" <- w16
  "Compile Folder" <- w15
  "MailBody" <- w13
  "Compile FPGA-Target" <- w12
  "コンパイル中" <- w11
  "Log" <- w9
  "smtp error msg" <- w4
